vi "Func-데이터 타입 변환-32비트 정수 실수.vi"() -> ()   [LabVIEW 2015]
panel:
  out "INT32U 4":u32 format="%08x"
  in  "INT32U 3":u32 format="%08x"
  out "FP32 3":sgl format="%#_10g"
  out "FP32 2":sgl format="%#_10g"
  in  "INT32U 2":u32 format="%08d"
  out "INT32U":u32 format="%08d"
  in  "FP32":sgl format="%#_10g"
  # "실수형을 4바이트로"
  # "4바이트를 실수형으로"
  # "4바이트를 실수형으로"
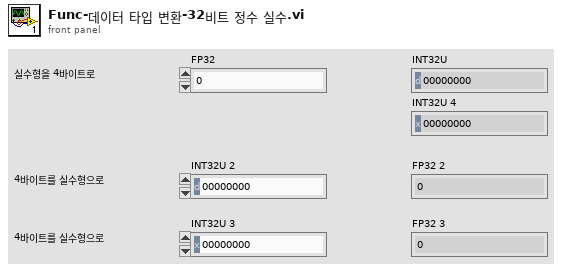
[diagram p1: front panel]
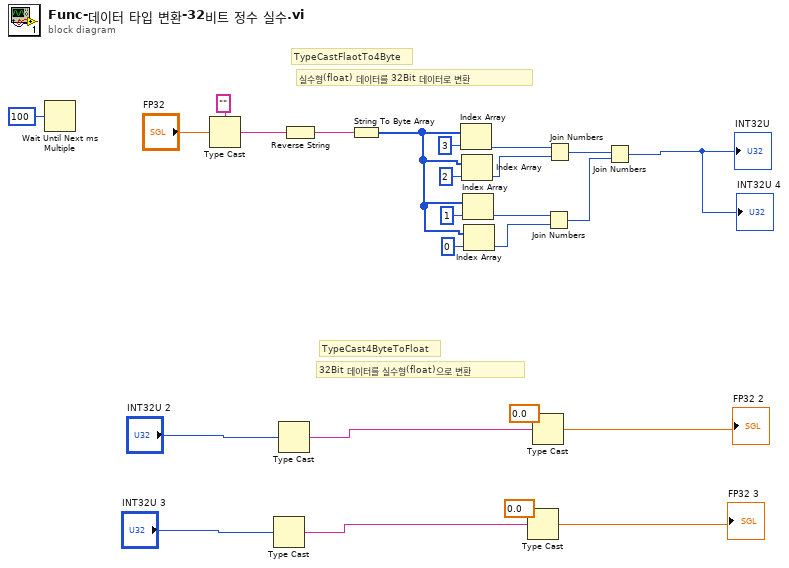
[diagram p0: block diagram]
diagram:
  # "32Bit 데이터를 실수형(float)으로 변환"
  # "실수형(float) 데이터를 32Bit 데이터로 변환"
  # "TypeCastFlaotTo4Byte"
  # "TypeCast4ByteToFloat"
  n1 = Wait Until Next ms Multiple(millisecond multiple=u32 100 ("ms 배수")) -> ()  [unwired: 1 out]
  n2 = Type Cast(type="" ("타입"), x="FP32") -> (*(type *) &x=w25:string)
  n3 = Type Cast(x="INT32U 3") -> (*(type *) &x=w5:string)  [unwired: 1 in]
  n4 = Type Cast(x="INT32U 2") -> (*(type *) &x=w7:string)  [unwired: 1 in]
  n5 = Reverse String(1:w25) -> (0:w23:string)
  n6 = String To Byte Array(string=w23) -> (unsigned byte array=w18:u8[])
  n7 = Index Array(array=w18, index=3 ("인덱스")) -> (element=w17:u8)
  n8 = Index Array(array=w18, index=2 ("인덱스")) -> (element=w16:u8)
  n9 = Index Array(array=w18, index=1 ("인덱스")) -> (element=w15:u8)
  n10 = Index Array(array=w18, index=0 ("인덱스")) -> (element=w14:u8)
  n11 = Type Cast(type=sgl 0.0, x=w5) -> (*(type *) &x=→"FP32 3":sgl)
  n12 = Type Cast(type=sgl 0.0, x=w7) -> (*(type *) &x=→"FP32 2":sgl)
  n13 = Join Numbers(hi=w15, lo=w14) -> ((hi.lo)=w12:u16)
  n14 = Join Numbers(hi=w17, lo=w16) -> ((hi.lo)=w13:u16)
  n15 = Join Numbers(hi=w13, lo=w12) -> ((hi.lo)=→"INT32U" →"INT32U 4":u32)
